vi "AutoSetRLEDemands.vi"(8 "error in (no error)":errorcluster, 9 "SetExtendPositonDemand(in)":dbl, 10 "SetLIftPostionDemand(d)":dbl, 11 "SetRotatePostionDemand(d)":dbl) -> (0 "error out":errorcluster)   [LabVIEW 2020]
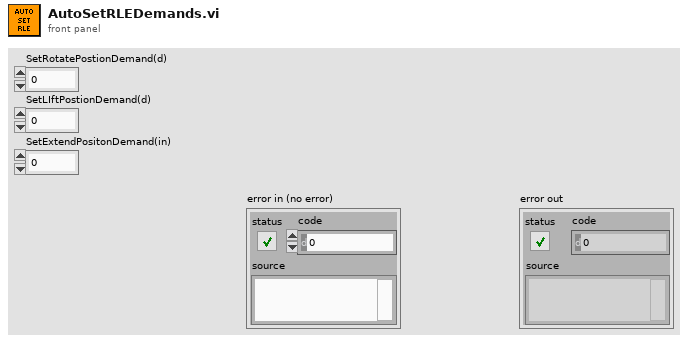
[diagram p1: front panel]
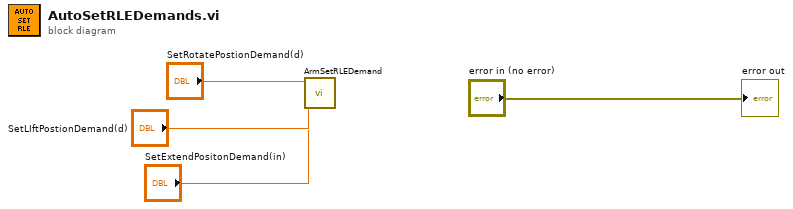
[diagram p0: block diagram]
diagram:
  n1 = call "ArmSetRLEDemand.vi"("SetExtendPositonDemand(in)"="SetExtendPositonDemand(in)", "SetLIftPostionDemand(d)"="SetLIftPostionDemand(d)", "SetRotatePostionDemand(d)"="SetRotatePostionDemand(d)") -> ()  [unwired: 9 in]
  "error out" <- "error in (no error)"
